vi "Fire Transient.vi"(8 "error in":errorcluster, 10 "AI Connection In":T1, 11 "Carrier Connection In":T1={"Description"="", "Address"="", "Port"=0, "timeout (ms)"=5000, "Termination Character"="\n", "TCP Connection Reference"=refnum, "Open Connection"=FALSE}) -> (0 "error out":errorcluster, 2 "AI Connection Out":T1, 3 "Carrier Connection Out":T1)   [LabVIEW 2017, in "DTACQ - Network Enabled Device Driver.lvlib"]
doc: "Arms and fires a transient shot. Waits until data is ready for downoad, before exiting the VI."
uses:
  DTACQ - Network Enabled Device Driver.lvlib
  Communications/Typedefs/DTACQ Connection Data--Cluster.ctl
  Communications/Communications Library.lvlib
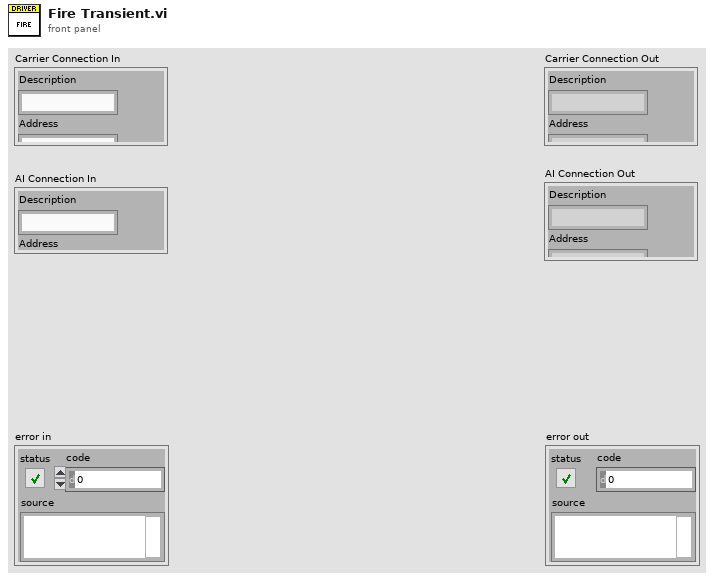
[diagram p1: front panel]
types:
  T1 = typedef "Communications Library.lvlib/DTACQ Connection Data--Cluster.ctl" = cluster{"Description":string, "Address":string, "Port":u16, "timeout (ms)":i32, "Termination Character":string, "TCP Connection Reference":refnum<k5>, "Open Connection":bool}
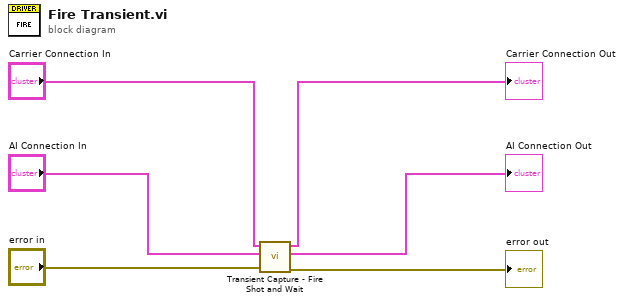
[diagram p0: block diagram]
diagram:
  n1 = call "Transient Capture - Fire Shot and Wait.vi"("error in"="error in", "Carrier Connection In"="AI Connection In", "AI Connection In"="Carrier Connection In") -> ("error out"=→"error out":errorcluster, "Carrier Connection Out"=→"AI Connection Out":T1, "AI Connection Out"=→"Carrier Connection Out":T1)  [unwired: 6 in]
